vi "SPI Read.vi"(0 "handle":u32, 1 "options":u32, 7 "sizeToTransfer":u32, 11 "error in (no error)":errorcluster) -> (4 "handle out":u32, 6 "buffer out":string, 8 "function return":u32, 10 "sizeTransfered out":u32, 15 "error out":errorcluster)   [LabVIEW 2018, in "libMPSSE-SPI.lvlib"]
doc: "FTDI_API FT_STATUS SPI_Read(FT_HANDLE handle, uint8 *buffer,\n uint32 sizeToTransfer, uint32 *sizeTransfered, uint32 options);"
uses:
  libMPSSE-SPI.lvlib
  dll/libMPSSE.dll
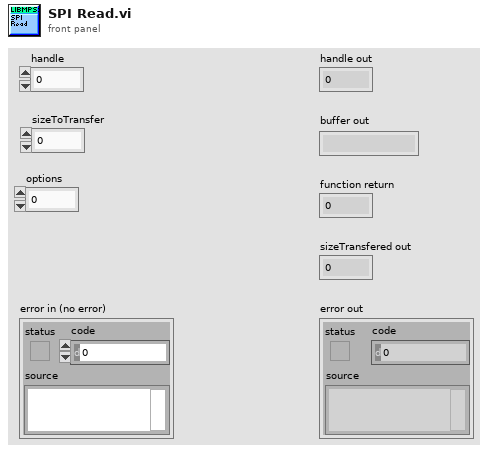
[diagram p1: front panel]
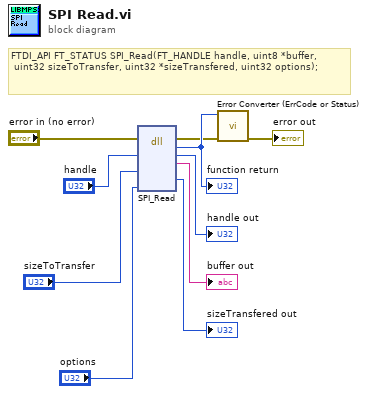
[diagram p0: block diagram]
diagram:
  # "FTDI_API FT_STATUS SPI_Read(FT_HANDLE handle, uint8 *buffer,\n\tuint32 sizeToTransfer, uint32 *sizeTransfered, uint32 options);"
  n1 = dll-call lib="D:/LABVIEW/Examples - 32bit/FTDI/libMPSSE-SPI-LabVIEW-master SNA v3/dll/libMPSSE.*" fn="SPI_Read"(error in="error in (no error)", "handle"="handle", "sizeToTransfer"="sizeToTransfer", "options"="options") -> (error out=w2:errorcluster, "return type"=w10:u32, "handle"=→"handle out":u32, "buffer"=→"buffer out":string, "sizeTransfered"=→"sizeTransfered out":u32)  [unwired: 6 in, 1 out]
  "function return" <- w10
  n2 = call "Error Converter (ErrCode or Status).vi"("error in (no error)"=w2, "error code"=w10) -> ("error out"=→"error out":errorcluster)  [unwired: 9 in]
